vi "testParseNotReadingModifiedDataProperly(Case5788).vi"(8 "error in (no error)":errorcluster, 11 "reference in":refnum<class "EasyXML_XML_Subset_Source_Tests.lvclass">) -> (0 "error out":errorcluster, 3 "reference in":refnum<class "EasyXML_XML_Subset_Source_Tests.lvclass">)   [LabVIEW 2013, in "EasyXML_XML_Subset_Source_Tests.lvclass"]
uses:
  EasyXML_XML_Subset_Source_Tests.lvclass
  EasyXML_XML_Subset_Evaluations/EasyXML_XML_Subset_Evaluations.lvclass
panel:
  in  "sequence":T1={"version"=1.0, "test"="hello", "new feature"=0.0}
  out "sequence":T1
  in  "XML String":string="<sequence>\r\n  <version>1</version>\r\n  <test>hello</test>\r\n</sequence>"
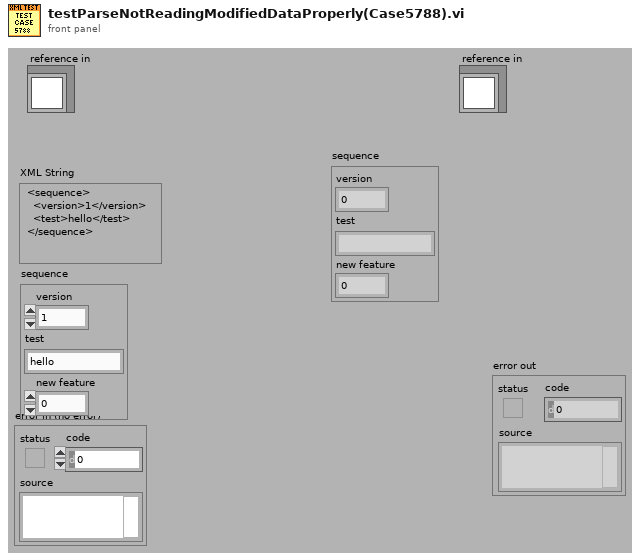
[diagram p1: front panel]
types:
  T1 = cluster{"version":dbl, "test":string, "new feature":dbl}
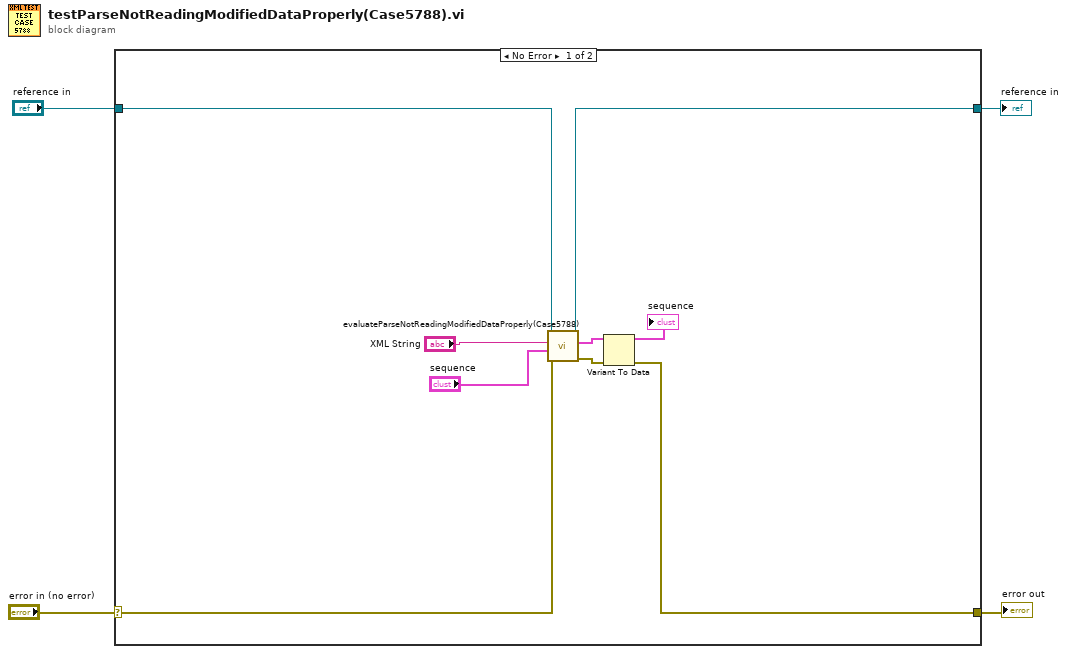
[diagram p0: block diagram]
diagram:
  n1 = case shown="No Error" "error in (no error)" {
    selector: "error in (no error)" -> [w11 w15]
    tunnel: [w5 w15] -> w3
    tunnel: [w12 w14] -> w1
    tunnel: "reference in" -> [w13 w14]
    frame No Error {
      n2 = call "evaluateParseNotReadingModifiedDataProperly(Case5788).vi"("error in (no error)"=w11, "sequence"="sequence", "XML String"="XML String", "reference in"=w13) -> ("error out"=w6:errorcluster, "sequence"=w9:T1, "reference in"=w12:refnum<class "EasyXML_XML_Subset_Source_Tests.lvclass">)  [unwired: 5 in]
      n3 = Variant To Data(error in=w6, Variant=w9) -> (data=→"sequence":T1, error out=w5:errorcluster)  [unwired: 1 in]
    }
    frame Error {
    }
  }
  "error out" <- w3
  "reference in" <- w1
